vi "get_com_port.vi"(8 "error in (no error)":errorcluster, 11 "LightSourceMH110124MaiTai in":refnum<class "LightSourceMH110124MaiTai.lvclass">) -> (0 "error out":errorcluster, 2 "comm port":refnum<visa-resource-name>, 3 "LightSourceMH110124MaiTai out":refnum<class "LightSourceMH110124MaiTai.lvclass">)   [LabVIEW 2010, in "LightSourceMH110124MaiTai.lvclass"]
uses:
  LightSourceMH110124MaiTai.lvclass
  LightSourceMH110124MaiTai.lvclass/LightSourceMH110124MaiTai.ctl
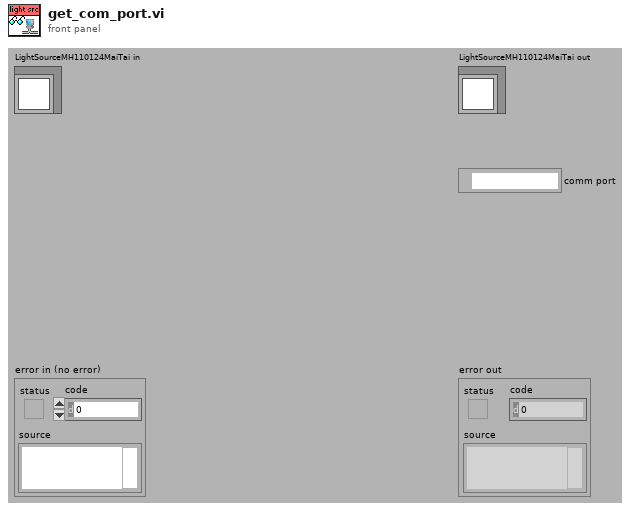
[diagram p1: front panel]
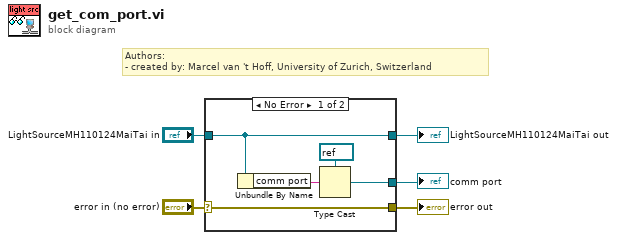
[diagram p0: block diagram]
diagram:
  # "Authors: \n- created by: Marcel van 't Hoff, University of Zurich, Switzerland"
  n1 = case shown="No Error" "error in (no error)" {
    selector: "error in (no error)" -> [w10 w12]
    tunnel: [w10 w12] -> w4
    tunnel: [w9 w11] -> w2
    tunnel: "LightSourceMH110124MaiTai in" -> [w9 w11]
    tunnel: [w7 _] -> w1
    frame No Error {
      n2 = Unbundle By Name(w9) -> ("comm port"=w8:string)
      n3 = Type Cast(type=refnum<visa-resource-name> refnum ("comm port"), x=w8) -> (*(type *) &x=w7:refnum<visa-resource-name>)
    }
    frame Error {
    }
  }
  "error out" <- w4
  "LightSourceMH110124MaiTai out" <- w2
  "comm port" <- w1
